vi "Get Protection Signals.vi"(10 "Frame.Data in":dbl[](array[numeric]), 11 "Protection Configuration":T1 {"CRC Channels"."Data Type" items=["Signed", "Unsigned", "IEEE Float"]}) -> (2 "Frame.Data out":dbl[](array[numeric]), 3 "Protection Configuration out":T1 {"CRC Channels"."Data Type" items=["Signed", "Unsigned", "IEEE Float"]})   [LabVIEW 2019, in "Protection and Counter Support Engine.lvlib"]
uses:
  Protection and Counter Support Engine.lvlib
  Types/RT Protection Configuration.ctl
  Shared/Types/Protection Type.ctl
  Shared/Types/XNET Signal Configuration.ctl
  Shared/Protection and Counter Support Shared.lvlib
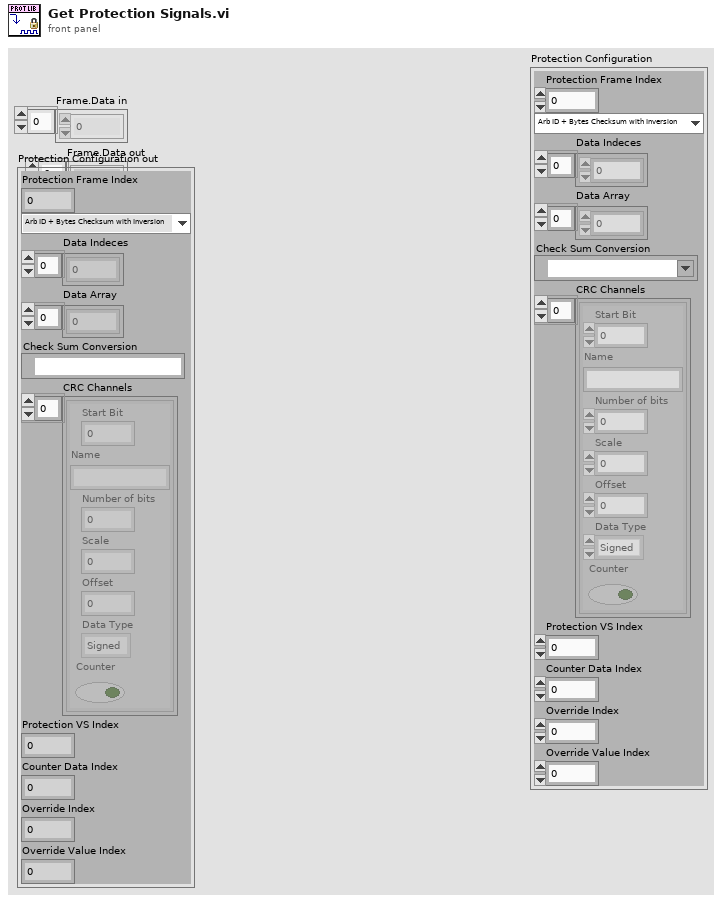
[diagram p1: front panel]
types:
  T1 = typedef "Protection and Counter Support Engine.lvlib/RT Protection Configuration.ctl" = cluster{"Protection Frame Index":i32, "Protection Type":T2, "Data Indeces":i32[], "Data Array":dbl[], "Check Sum Conversion":refnum<k21>, "CRC Channels":T3[], "Protection VS Index":i32, "Counter Data Index":i32, "Override Index":i32, "Override Value Index":i32}
  T2 = typedef "Protection and Counter Support Shared.lvlib/Protection Type.ctl" = enum16{"Arb ID + Bytes Checksum with Inversion", "Arb ID + Bytes CRC with Inversion", "Reversed Raw Signal Checksum with Inversion", "Concatenated Two's Compliment"}
  T3 = typedef "Protection and Counter Support Shared.lvlib/XNET Signal Configuration.ctl" = cluster{"Start Bit":i32, "Name":string, "Number of bits":i32, "Scale":dbl, "Offset":dbl, "Data Type":u32, "Counter":bool}
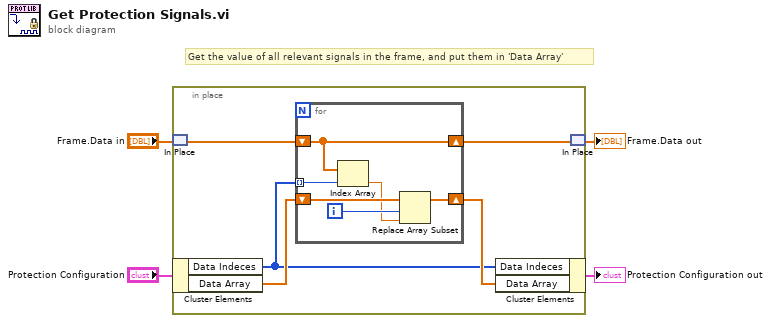
[diagram p0: block diagram]
diagram:
  # "Get the value of all relevant signals in the frame, and put them in 'Data Array'"
  n1 = in-place {
    n2 = in-place-match #1("Frame.Data in") -> (w6:dbl[])
    n3 = in-place-cluster #2("Protection Configuration") -> ("Data Indeces"=w7:i32[], "Data Array"=w9:dbl[])
    n4 = for {
      shift-right: [w14] -> w5
      shift-left: w6 -> [w14]
      tunnel: w7 -> [w15] mode=indexing
      shift-right: [w10] -> w8
      shift-left: w9 -> [w13]
      i -> [w12]
      n5 = Index Array(array=w14, index=w15) -> (element=w11:dbl)
      n6 = Replace Array Subset(array=w13, new element=w11, index=w12) -> (w10:dbl[])
    }
    n7 = in-place-cluster #2("Data Indeces"=w7, "Data Array"=w8) -> (→"Protection Configuration out":T1)
    n8 = in-place-match #1(w5) -> (→"Frame.Data out":dbl[])
  }
